vi "BRAM_WriteScore.vi"(1 "Data":fxp<+,4,4>, 4 "Address":i16, 8 "Player":u8) -> ()   [LabVIEW 2018]
uses:
  <vilib>/rvi/Memory/Memory_Emulation/nirvimemoryFastEmulation.vi
  <vilib>/rvi/Memory/Memory_Emulation/nirvimemoryEmulation.vi
  <vilib>/rvi/Emulation/niFpgaEmulationIsFPGAContextNoSignature.vi
  <vilib>/rvi/DataTransferAndStorage/Container/Common/niFpgaContainerGetUniqueNameForEmu.vi
  <vilib>/rvi/Emulation/niFpgaProcessEmulError.vi
  <vilib>/rvi/Emulation/niFpgaSctlEmulationGetInTimedLoop.vi
  <vilib>/rvi/errors/nirviReportUnexpectedCaseInternalError (U32).vi
  <vilib>/rvi/DataTransferAndStorage/Container/XNode/niFpgaContainer.xnode
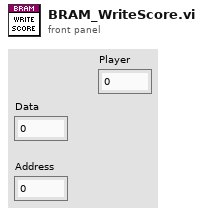
[diagram p1: front panel]
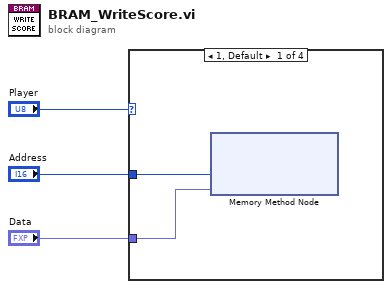
[diagram p0: block diagram]
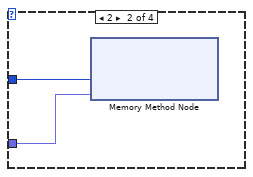
[diagram p2: hidden frame]
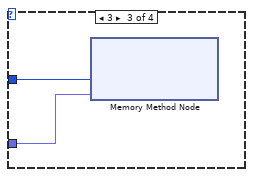
[diagram p3: hidden frame]
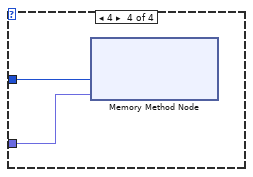
[diagram p4: hidden frame]
diagram:
  n1 = case shown="1, Default" "Player" {
    tunnel: "Address" -> [w5 w7 w9 w11]
    tunnel: "Data" -> [w4 w6 w8 w10]
    frame 1, Default {
      n2 = xnode ("Memory Method Node")("Address"=w5, "Data"=w4) -> ()  [unwired: 1 in, 1 out]
    }
    frame 2 {
      n3 = xnode ("Memory Method Node")("Address"=w7, "Data"=w6) -> ()  [unwired: 1 in, 1 out]
    }
    frame 3 {
      n4 = xnode ("Memory Method Node")("Address"=w9, "Data"=w8) -> ()  [unwired: 1 in, 1 out]
    }
    frame 4 {
      n5 = xnode ("Memory Method Node")("Address"=w11, "Data"=w10) -> ()  [unwired: 1 in, 1 out]
    }
  }
